vi "transUkToDof.vi"(8 "error in (no error)":errorcluster, 10 "uk Array":dbl[](array[numeric]), 11 "ZTAAC in":refnum<class "ZTAAC.lvclass">) -> (0 "error out":errorcluster, 2 "State in DOF":dbl[](array[numeric]), 3 "ZTAAC out":refnum<class "ZTAAC.lvclass">)   [LabVIEW 2016, in "OfcFunc.lvlib" / "ZTAAC.lvclass"]
doc: "Transform uk to the degree of freedom (DOF) based on the index array of DOF."
uses:
  ZTAAC.lvclass
  ZTAAC.lvclass/ZTAAC.ctl
  OptStateEsti/OptStateEsti.lvclass
  OptCtrl/OptCtrl.lvclass
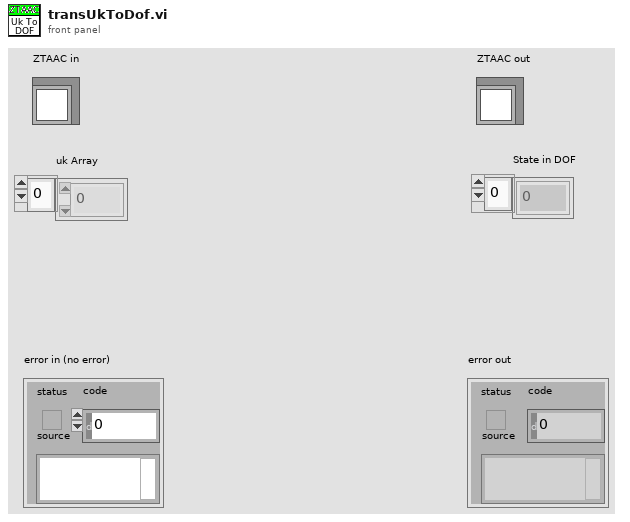
[diagram p1: front panel]
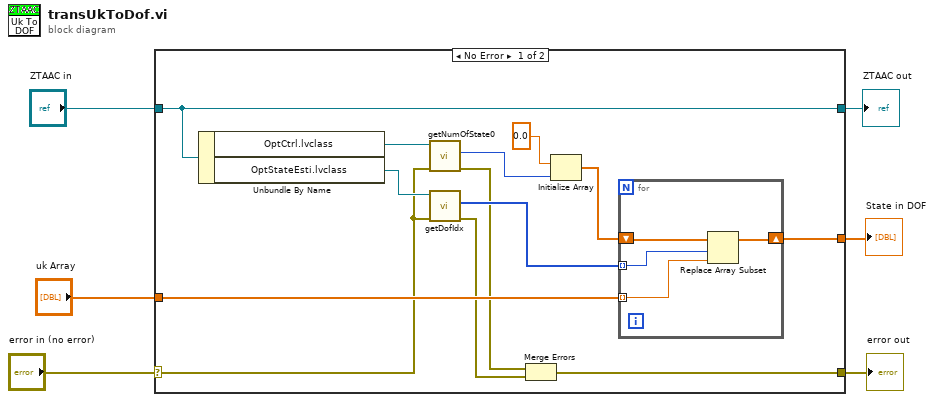
[diagram p0: block diagram]
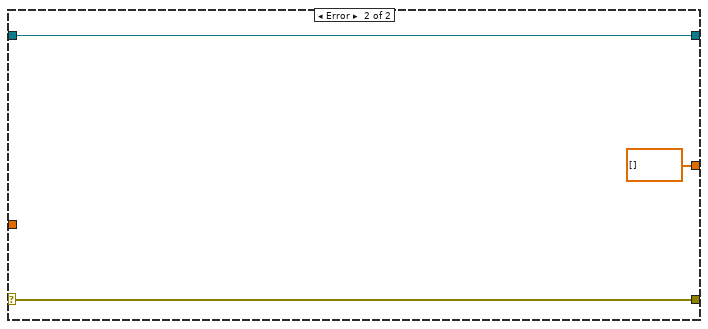
[diagram p2: hidden frame]
diagram:
  n1 = case shown="No Error" "error in (no error)" {
    selector: "error in (no error)" -> [w10 w26]
    tunnel: [w7 w26] -> w5
    tunnel: [w19 w25] -> w3
    tunnel: "ZTAAC in" -> [w19 w25]
    tunnel: "uk Array" -> [w12 _]
    tunnel: [w11 dbl[] []] -> w1
    frame No Error {
      n2 = Unbundle By Name(w19) -> ("OptCtrl.lvclass"=w18:refnum<class "OptCtrl.lvclass">, "OptStateEsti.lvclass"=w17:refnum<class "OptStateEsti.lvclass">)
      n3 = call "getNumOfState0.vi"("error in (no error)"=w10, "OptCtrl in"=w18) -> ("error out"=w9:errorcluster, "Num of State 0"=w16:i32)  [unwired: 7 in, 1 out]
      n4 = call "getDofIdx.vi"("error in (no error)"=w10, "OptStateEsti in"=w17) -> ("error out"=w8:errorcluster, "dofIdx"=w14:i32[])  [unwired: 7 in, 1 out]
      n5 = Merge Errors(w9, w8) -> (w7:errorcluster)
      n6 = Initialize Array(0.0 ("element"), w16) -> (w13:dbl[])
      n7 = for {
        tunnel: w14 -> [w21] mode=indexing
        shift-right: [w22] -> w11
        shift-left: w13 -> [w23]
        tunnel: w12 -> [w20] mode=indexing
        n8 = Replace Array Subset(array=w23, new element=w20, index=w21) -> (w22:dbl[])
      }
    }
    frame Error {
    }
  }
  "error out" <- w5
  "ZTAAC out" <- w3
  "State in DOF" <- w1
